vi "UnloadAction.vi"(8 "error in (no error)":errorcluster caption="entrée d'erreur (pas d'erreur)", 11 "Tools In":refnum<class "ThorPM100A.lvclass"> caption="DNL_LabVIEW Object in") -> (0 "error out":errorcluster caption="sortie d'erreur", 3 "Tools Out":refnum<class "ThorPM100A.lvclass"> caption="DNL_LabVIEW Object out")   [LabVIEW 2019, in "ThorPM100A.lvclass"]
uses:
  ThorPM100A.lvclass
  C:/Programmes Labview/LabScanV1A/DevicesClass/BaseDevice/BaseDevice.lvclass
  BaseDevice/BaseDevice.lvclass
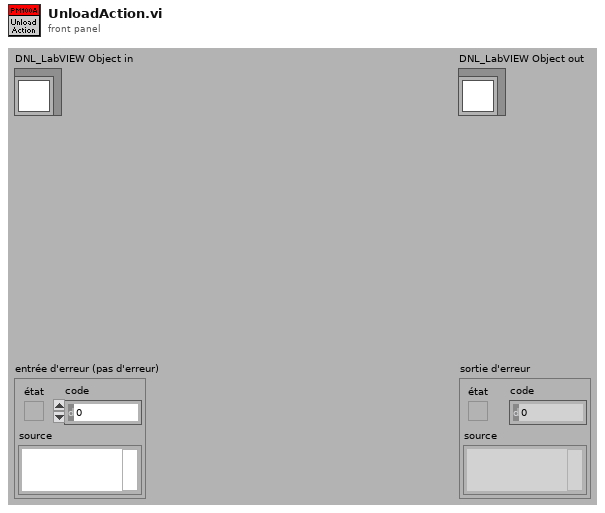
[diagram p1: front panel]
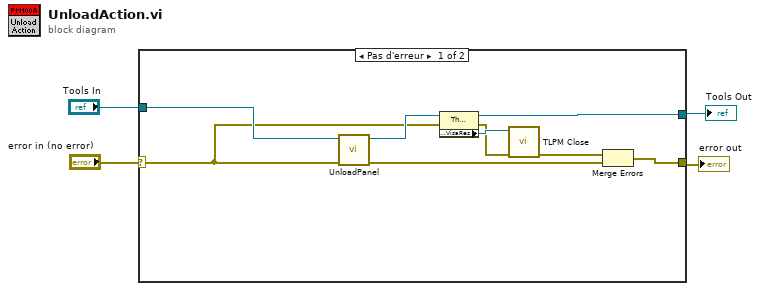
[diagram p0: block diagram]
diagram:
  n1 = case shown="Pas d'erreur" "error in (no error)" {
    selector: "error in (no error)" -> [w8 w14]
    tunnel: [w6 w14] -> w3
    tunnel: [w10 w15] -> w2
    tunnel: "Tools In" -> [w11 w15]
    frame No Error {
      n2 = call "UnloadPanel.vi"("error in (no error)"=w8, "Device en entrée"=w11) -> ("error out"=w13:errorcluster, "Device en sortie"=w12:refnum<class "ThorPM100A.lvclass">)  [unwired: 8 in]
      n3 = property class="ThorPM100A.lvclass"(reference=w12, error in=w8) -> (reference out=w10:refnum<class "ThorPM100A.lvclass">, error out=w7:errorcluster, "Accessor:VisaRes"=w9:refnum<visa-resource-name>)
      n4 = call <instrlib>:"TLPM Close.vi"("error in (no error)"=w7, "instrument handle"=w9) -> ("error out"=w5:errorcluster)  [unwired: 9 in]
      n5 = Merge Errors(w5, w13) -> (w6:errorcluster)
    }
    frame Error {
    }
  }
  "error out" <- w3
  "Tools Out" <- w2
